vi "find_rects.vi"(5 "shrinkFactor":i32=1, 6 "Field of View":cluster{"fieldOfViewX":sgl, "fieldOfViewY":sgl}, 8 "error in":errorcluster, 10 "find_patches parameters":T2, 11 "Image":T3) -> (0 "error out":errorcluster, 2 "rects":T1(array[cluster]))   [LabVIEW 2024, in "Vision.lvlib"]
uses:
  Vision.lvlib
  <vilib>/vision/Image Controls.llb/IMAQ Image.ctl
  find_rects_parameters.ctl
  bin/PatternRecognition.dll
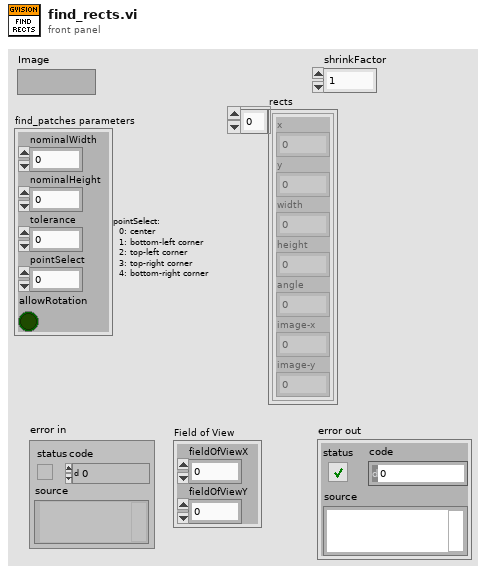
[diagram p1: front panel]
types:
  T1 = cluster{"x":dbl, "y":dbl, "width":dbl, "height":dbl, "angle":dbl, "image-x":dbl, "image-y":dbl}[]
  T2 = typedef "Vision.lvlib/find_rects_parameters.ctl" = cluster{"nominalWidth":sgl, "nominalHeight":sgl, "tolerance":sgl, "pointSelect":sgl, "allowRotation":bool}
  T3 = typedef "IMAQ Image.ctl" = refnum<image>
  T4 = enum32{"Map Pixel Pointer", "Unmap Pixel Pointer", "Get Pixels Infos"}
  T5 = cluster{"x":dbl, "y":dbl, "width":dbl, "height":dbl, "angle":dbl, "image-x":dbl, "image-y":dbl}
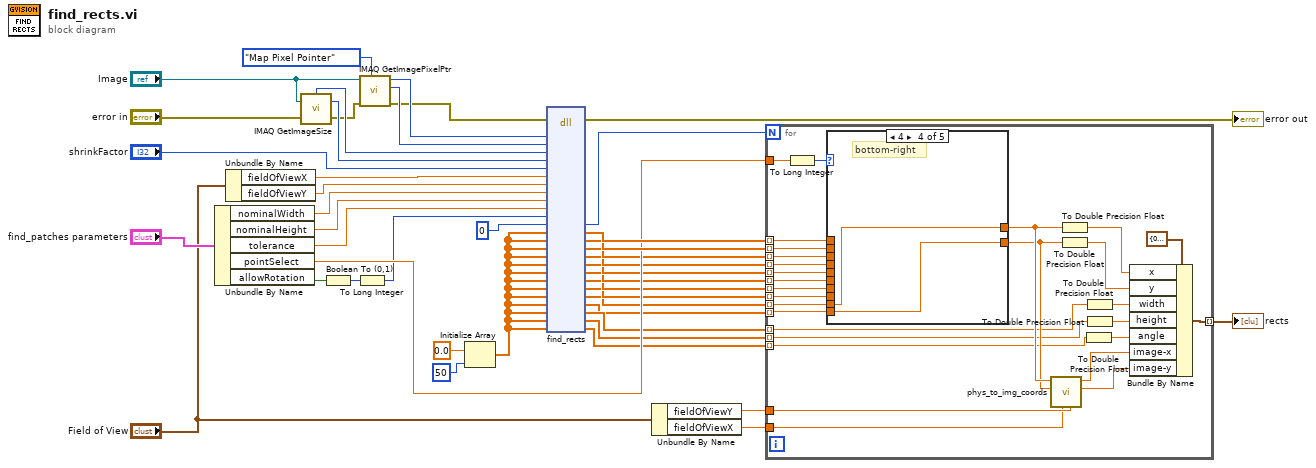
[diagram p0: block diagram]
diagram:
  n1 = Unbundle By Name("find_patches parameters") -> ("nominalWidth"=w27:sgl, "nominalHeight"=w26:sgl, "tolerance"=w25:sgl, "pointSelect"=w16:sgl, "allowRotation"=w2:bool)
  n2 = Unbundle By Name("Field of View") -> ("fieldOfViewX"=w30:sgl, "fieldOfViewY"=w29:sgl)
  n3 = call "IMAQ GetImageSize"("Image"="Image", "error in (no error)"="error in") -> ("Y Resolution"=w39:i32, "X Resolution"=w40:i32, "error out"=w33:errorcluster)  [unwired: 2 in]
  n4 = Boolean To (0,1)(Boolean=w2) -> (0, 1=w4:i16)
  n5 = To Long Integer(number=w4) -> (32bit integer=w3:i32)
  n6 = call "IMAQ GetImagePixelPtr"("Function"=T4."Map Pixel Pointer", "error in (no error)"=w33, "Image"="Image") -> ("error out"=w32:errorcluster, "LineWidth(Pixels)"=w41:i32, "Pixel Pointer out"=w42:u64)  [unwired: 3 in, 3 out]
  n7 = Initialize Array(sgl 0.0 ("element"), 50 ("dimension size")) -> (w1:sgl[])
  n8 = dll-call lib="C:/Users/cfang/Desktop/nebraska-silicon-lab/pixel-gantry-control/Gantry/Shared Components/bin/PatternRecognition.dll" fn="find_rects"(error in=w32, "imgPtr"=w42, "imgLineWidth"=w41, "imgWidth"=w40, "imgHeight"=w39, "shrinkFactor"="shrinkFactor", "fieldOfViewX"=w30, "fieldOfViewY"=w29, "nominalWidth"=w27, "nominalHeight"=w26, "tolerance"=w25, "allowRotation"=w3, "Nrects"=0, "rectXCenters"=w1, "rectYCenters"=w1, "rectXBLCorners"=w1, "rectYBLCorners"=w1, "rectXTLCorners"=w1, "rectYTLCorners"=w1, "rectXTRCorners"=w1, "rectYTRCorners"=w1, "rectXBRCorners"=w1, "rectYBRCorners"=w1, "rectWidths"=w1, "rectHeights"=w1, "rectAngles"=w1) -> (error out=→"error out":errorcluster, "Nrects"=w21:i32, "rectXCenters"=w20:sgl[], "rectYCenters"=w19:sgl[], "rectXBLCorners"=w12:sgl[], "rectYBLCorners"=w11:sgl[], "rectXTLCorners"=w10:sgl[], "rectYTLCorners"=w9:sgl[], "rectXTRCorners"=w8:sgl[], "rectYTRCorners"=w7:sgl[], "rectXBRCorners"=w6:sgl[], "rectYBRCorners"=w5:sgl[], "rectWidths"=w13:sgl[], "rectHeights"=w14:sgl[], "rectAngles"=w15:sgl[])  [unwired: 14 in, 1 out]
  n9 = Unbundle By Name("Field of View") -> ("fieldOfViewY"=w24:sgl, "fieldOfViewX"=w23:sgl)
  n10 = for {
    N: w21 -> [_]
    tunnel: w20 -> [w62] mode=indexing
    tunnel: w19 -> [w61] mode=indexing
    tunnel: [w71] -> w17 mode=indexing
    tunnel: w24 -> [w58]
    tunnel: w23 -> [w57]
    tunnel: w14 -> [w54] mode=indexing
    tunnel: w16 -> [w55]
    tunnel: w15 -> [w53] mode=indexing
    tunnel: w13 -> [w52] mode=indexing
    tunnel: w12 -> [w51] mode=indexing
    tunnel: w11 -> [w50] mode=indexing
    tunnel: w10 -> [w49] mode=indexing
    tunnel: w9 -> [w48] mode=indexing
    tunnel: w8 -> [w47] mode=indexing
    tunnel: w7 -> [w46] mode=indexing
    tunnel: w6 -> [w45] mode=indexing
    tunnel: w5 -> [w44] mode=indexing
    n11 = To Long Integer(number=w55) -> (32bit integer=w56:i32)
    n12 = case shown="4" w56 {
      tunnel: w62 -> [_ _ _ _ w81]
      tunnel: w61 -> [_ _ _ _ w80]
      tunnel: [w73 w75 w77 w79 w81] -> w60
      tunnel: [w72 w74 w76 w78 w80] -> w59
      tunnel: w51 -> [w73 _ _ _ _]
      tunnel: w50 -> [w72 _ _ _ _]
      tunnel: w49 -> [_ w75 _ _ _]
      tunnel: w48 -> [_ w74 _ _ _]
      tunnel: w47 -> [_ _ w77 _ _]
      tunnel: w46 -> [_ _ w76 _ _]
      tunnel: w45 -> [_ _ _ w79 _]
      tunnel: w44 -> [_ _ _ w78 _]
      frame 1 {
        # "bottom-left"
      }
      frame 2 {
        # "top-left"
      }
      frame 3 {
        # "top-right"
      }
      frame 4 {
        # "bottom-right"
      }
      frame 0, Default {
        # "center"
      }
    }
    n13 = call "phys_to_img_coords.vi"("fov_y"=w58, "fov_x"=w57, "y"=w59, "x"=w60) -> ("image_y"=w66:dbl, "image_x"=w67:dbl)  [unwired: 6 in]
    n14 = To Double Precision Float(number=w60) -> (double precision float=w70:dbl)
    n15 = To Double Precision Float(number=w59) -> (double precision float=w69:dbl)
    n16 = To Double Precision Float(number=w53) -> (double precision float=w63:dbl)
    n17 = To Double Precision Float(number=w52) -> (double precision float=w68:dbl)
    n18 = To Double Precision Float(number=w54) -> (double precision float=w65:dbl)
    n19 = Bundle By Name(cluster=T5 {"x"=0.0, "y"=0.0, "width"=0.0, "height"=0.0, "angle"=0.0, "image-x"=0.0, "image-y"=0.0}, "x"=w70, "y"=w69, "width"=w68, "height"=w65, "angle"=w63, "image-x"=w67, "image-y"=w66) -> (w71:T5)
  }
  "rects" <- w17
